vi "build_data_arrays.vi"(7 "last_test":dbl[](array[numeric]), 10 "Test":T1, 11 "test_data in":T2) -> (3 "test_data out":T2)   [LabVIEW 2024]
uses:
  test_data--cluster.ctl
  Labs/Encoding Lab/Tests/tests--enum.ctl
  <vilib>/Analysis/NI_AALBase.lvlib
  Labs/Encoding Lab/EncodingTester.lvlib
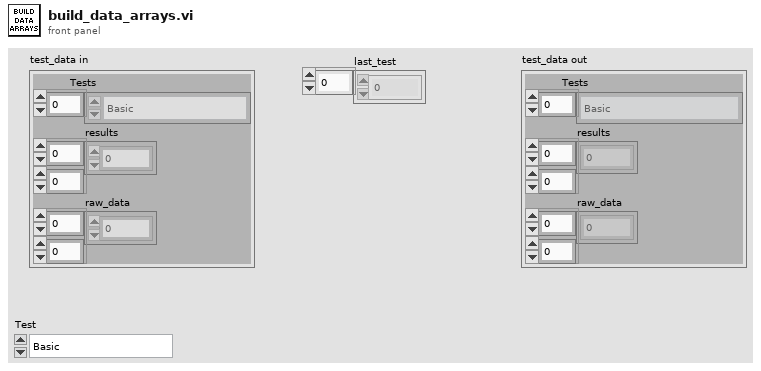
[diagram p1: front panel]
types:
  T1 = typedef "EncodingTester.lvlib/tests--enum.ctl" = enum16{"Basic", "Pre-Allocated", "Packet-Type Case", "No IPE"}
  T2 = typedef "test_data--cluster.ctl" = cluster{"Tests":T1[], "results":dbl[][], "raw_data":dbl[][]}
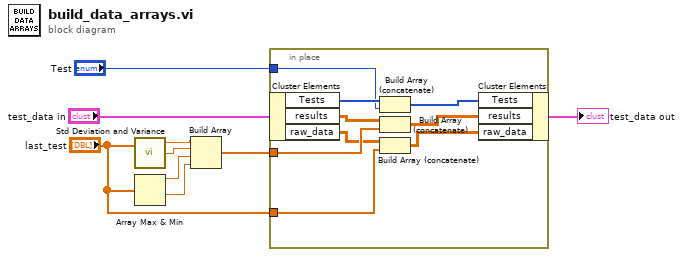
[diagram p0: block diagram]
diagram:
  n1 = call <vilib>:"Std Deviation and Variance.vi"("X"="last_test") -> ("mean"=w9:dbl, "standard deviation"=w8:dbl)  [unwired: 1 in, 1 out]
  n2 = Array Max & Min(array="last_test") -> (max value=w7:dbl, min value=w6:dbl)  [unwired: 2 out]
  n3 = Build Array(w9, w8, w7, w6) -> (w2:dbl[])
  n4 = in-place {
    in-place-border: "Test" -> [w17]
    in-place-border: w2 -> [w16]
    in-place-border: "last_test" -> [w13]
    n5 = in-place-cluster #1("test_data in") -> ("Tests"=w18:T1[], "results"=w15:dbl[][], "raw_data"=w14:dbl[][])
    n6 = Build Array (concatenate)(w18, w17) -> (w10:T1[])
    n7 = Build Array (concatenate)(w15, w16) -> (w11:dbl[][])
    n8 = Build Array (concatenate)(w14, w13) -> (w12:dbl[][])
    n9 = in-place-cluster #1("Tests"=w10, "results"=w11, "raw_data"=w12) -> (→"test_data out":T2)
  }
